vi "ep_Simulate Flicker.vi"(0 "amplitude RMS [V]":dbl=230.0, 1 "init":bool, 5 "nominal frequency":enum16{"50 Hz", "60 Hz"}(ring), 7 "nominal sampling rate (Hz)":u16=9600, 9 "flicker frequency [Hz]":dbl=0.5, 11 "voltage fluctuation dV/V [%]":dbl=2.34, 12 "fluctuations shape":enum16{"sinusoidal", "rectangular"}(ring)) -> (4 "data":dbl[](array[numeric]), 6 "data multiplier":dbl[](array[numeric]))   [LabVIEW 2011]
uses:
  <vilib>/Analysis/NI_AALBase.lvlib
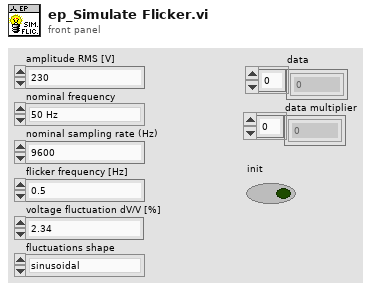
[diagram p1: front panel]
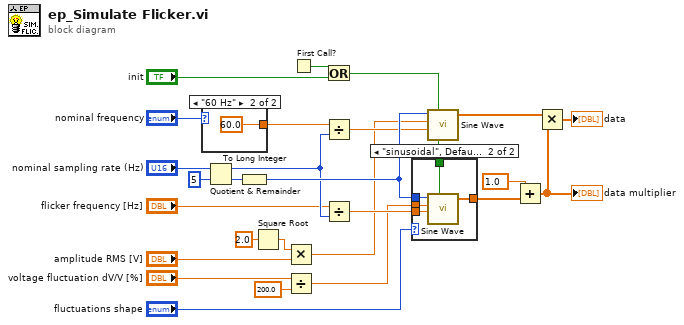
[diagram p0: block diagram]
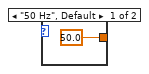
[diagram p2: hidden frame]
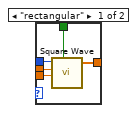
[diagram p3: hidden frame]
diagram:
  n1 = case shown="\"60 Hz\"" "nominal frequency" {
    tunnel: [50.0 ("y") 60.0 ("y")] -> w10
    frame "50 Hz", Default {
    }
    frame "60 Hz" {
    }
  }
  n2 = Quotient & Remainder(x="nominal sampling rate (Hz)", y=u16 5) -> (floor(x/y)=w18:u16)  [unwired: 1 out]
  n3 = To Long Integer(number=w18) -> (32bit integer=w16:i32)
  n4 = Square Root(x=2.0) -> (sqrt(x)=w25:dbl)
  n5 = Multiply(x=w25, y="amplitude RMS [V]") -> (x*y=w4:dbl)
  n6 = Divide(x="voltage fluctuation dV/V [%]", y=200.0 ("x")) -> (x/y=w5:dbl)
  n7 = First Call?() -> (First Call?: T/F=w2:bool)
  n8 = Or(x=w2, y="init") -> (x .or. y?=w1:bool)
  n9 = Divide(x=w10, y="nominal sampling rate (Hz)") -> (x/y=w9:dbl)
  n10 = Divide(x="flicker frequency [Hz]", y="nominal sampling rate (Hz)") -> (x/y=w6:dbl)
  n11 = case shown="\"sinusoidal\", Default" "fluctuations shape" {
    tunnel: w16 -> [w32 w37]
    tunnel: w5 -> [w31 w36]
    tunnel: [w29 w35] -> w14
    tunnel: w6 -> [w30 w34]
    tunnel: w1 -> [w28 w33]
    frame "rectangular" {
      n12 = call <vilib>:"Square Wave.vi"("samples"=w32, "reset phase"=w28, "amplitude"=w31, "frequency"=w30) -> ("square wave"=w29:dbl[])  [unwired: 2 in, 2 out]
    }
    frame "sinusoidal", Default {
      n13 = call <vilib>:"Sine Wave.vi"("samples"=w37, "amplitude"=w36, "frequency"=w34, "reset phase"=w33) -> ("sine wave"=w35:dbl[])  [unwired: 1 in, 2 out]
    }
  }
  n14 = call <vilib>:"Sine Wave.vi"("samples"=w16, "amplitude"=w4, "frequency"=w9, "reset phase"=w1) -> ("sine wave"=w12:dbl[])  [unwired: 1 in, 2 out]
  n15 = Add(x=1.0 ("Uref"), y=w14) -> (x+y=w22:dbl[])
  "data multiplier" <- w22
  n16 = Multiply(x=w12, y=w22) -> (x*y=→"data":dbl[])
